vi "emi_Graph Background.vi"(0 "Graph Refnum":refnum<vi>, 1 "Width(Screen)":i32=-1, 2 "Height(Screen)":i32=-1, 3 "Dark(Black)":u32(colorbox), 4 "Light(White)":u32(colorbox)=16448250, 5 "error in":errorcluster, 6 "Graphic Type(FlatColor)":T1, 7 "Grid(Black)":u32(colorbox)) -> (14 "Graph Refnum Out":refnum<vi>, 19 "error out":errorcluster)   [LabVIEW 2011]
doc: "Set the background graphic for a graph. \nNote that With and height must be bigger then the largest size for the graph. If left blank, a background the size of the screen is generated.\nGrid is the color of the Major grid lines.\n\nSupported graphs:\nXYGraph\nDigitalGraph\nWaveform Graph\nMixedSignal Graph\n\nOn other graphs the background color will simply be set to the light color.\n\nOn error: No action performed"
uses:
  0 - General/Graphix/Private/emi_List Of Graphix.ctl
  <vilib>/picture/picture.llb/imagedata.ctl
  0 - General/Graphix/emi_BW 8Bit image to Linear DuoTone.vi
  0 - General/Graphix/emi_Tile Gradient Image.vi
  <vilib>/picture/picture.llb/Draw Flattened Pixmap.vi
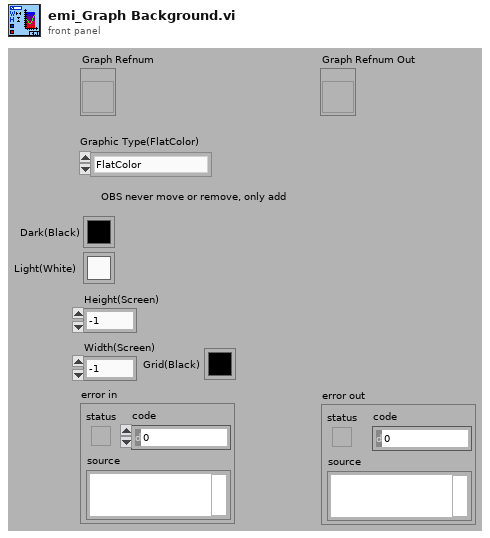
[diagram p1: front panel]
types:
  T1 = typedef "emi_List Of Graphix.ctl" = enum16{"FlatColor", "SharpGrad", "ShallowGrad", "GlasGradBord", "GlasGrad", "GlasGradBord 2"}
  T2 = typedef "imagedata.ctl" = cluster{"image type":i32, "image depth":i32, "image":u8[], "mask":u8[], "colors":u32[], "Rectangle":cluster{"left":i16, "top":i16, "right":i16, "bottom":i16}}
  T3 = typedef "LVRectTypeDef.ctl" = cluster{"left":i16, "top":i16, "right":i16, "bottom":i16}
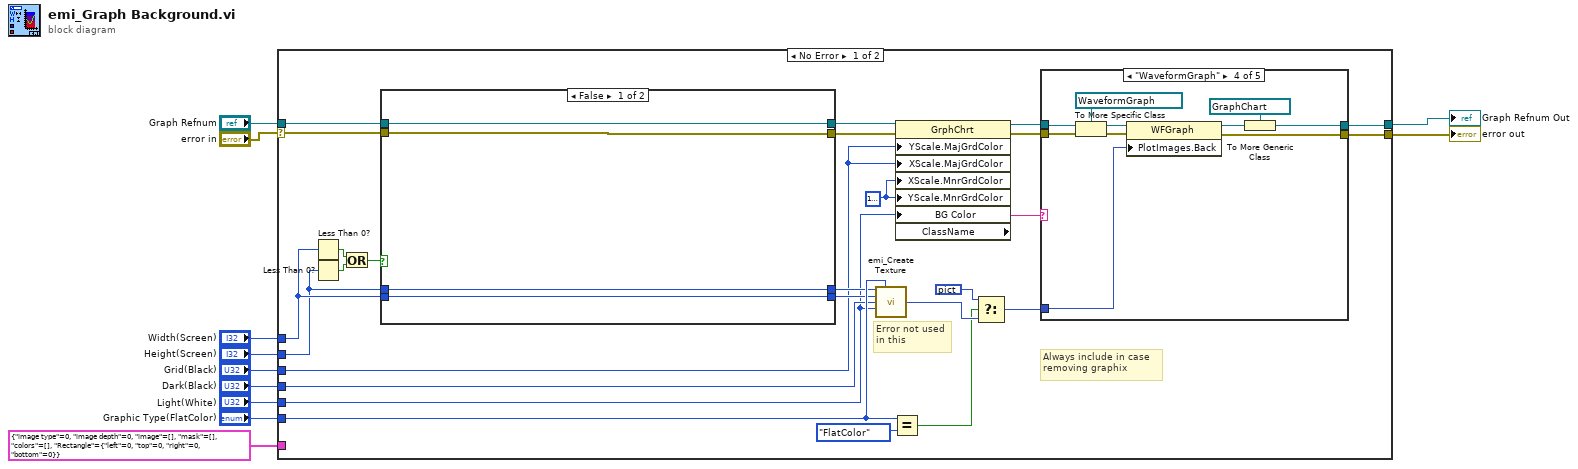
[diagram p0: block diagram]
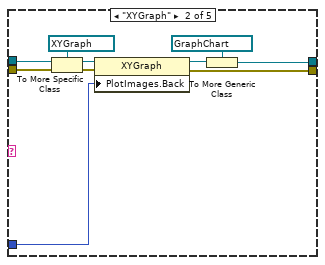
[diagram p3: hidden frame]
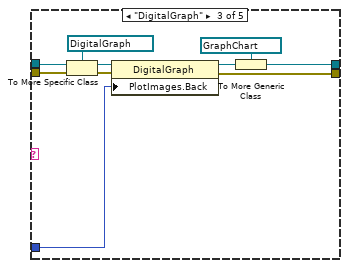
[diagram p4: hidden frame]
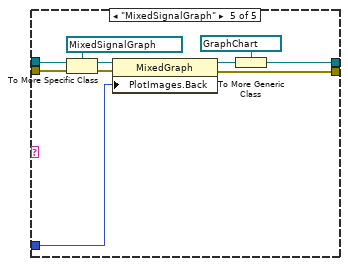
[diagram p5: hidden frame]
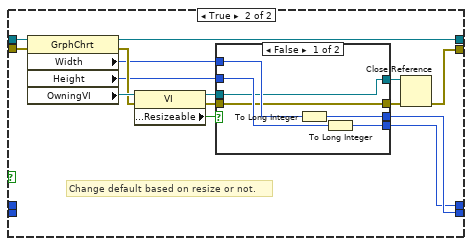
[diagram p6: hidden frame]
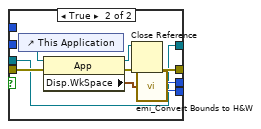
[diagram p7: hidden frame]
diagram:
  n1 = case shown="No Error" "error in" {
    selector: "error in" -> [w23 w115]
    tunnel: "Graphic Type(FlatColor)" -> [w36 _]
    tunnel: T2 {"image type"=0, "image depth"=0, "image"=[], "mask"=[], "colors"=[], "Rectangle"={"left"=0, "top"=0, "right"=0, "bottom"=0}} ("Image Data Out") -> [_ _]
    tunnel: "Graph Refnum" -> [w29 w114]
    tunnel: "Width(Screen)" -> [w26 _]
    tunnel: "Height(Screen)" -> [w25 _]
    tunnel: "Dark(Black)" -> [w20 _]
    tunnel: "Light(White)" -> [w13 _]
    tunnel: [w15 w115] -> w2
    tunnel: [w14 w114] -> w1
    tunnel: "Grid(Black)" -> [w12 _]
    frame No Error {
      w32 = u32 16777216 ("Light")
      # "Error not used\nin this"
      # "Always include in case\nremoving graphix"
      n2 = Less Than 0?(x=w26) -> (x < 0?=w30:bool)
      n3 = Less Than 0?(x=w25) -> (x < 0?=w31:bool)
      n4 = Or(x=w30, y=w31) -> (x .or. y?=w24:bool)
      n5 = case shown="False" w24 {
        tunnel: w29 -> [w83 w96]
        tunnel: [w83 w98] -> w28
        tunnel: w23 -> [w82 w97]
        tunnel: [w82 w86] -> w27
        tunnel: w26 -> [w80 _]
        tunnel: [w80 w89] -> w22
        tunnel: w25 -> [w81 _]
        tunnel: [w81 w88] -> w21
        frame False {
        }
        frame True {
          # "Change default based on resize or not."
          n6 = property class="GrphChrt"(reference=w96, error in=w97) -> (reference out=w98:refnum<vi>, error out=w94:errorcluster, "Width"=w91:u32, "Height"=w90:u32, "OwningVI"=w95:refnum<vi>)
          n7 = property class="VI"(reference=w95, error in=w94) -> (reference out=w85:refnum<vi>, error out=w93:errorcluster, "Front Panel.Resizeable"=w92:bool)
          n8 = case shown="False" w92 {
            tunnel: w93 -> [w102 w110]
            tunnel: [w102 w108] -> w87
            tunnel: w91 -> [w104 _]
            tunnel: w90 -> [w103 _]
            tunnel: [w100 w107] -> w89
            tunnel: [w99 w106] -> w88
            tunnel: w85 -> [w101 w105]
            tunnel: [w101 w105] -> w84
            frame False {
              n9 = To Long Integer(number=w104) -> (32bit integer=w100:i32)
              n10 = To Long Integer(number=w103) -> (32bit integer=w99:i32)
            }
            frame True {
              n11 = control-ref of="This Application"() -> (w109:refnum<vi>)
              n12 = property class="App"(reference=w109, error in=w110) -> (reference out=w112:refnum<vi>, error out=w113:errorcluster, "Disp.WkSpace"=w111:T3)
              n13 = Close Reference(reference=w112, error in (no error)=w113) -> (error out=w108:errorcluster)
              n14 = call "emi_Convert Bounds to H&W.vi"("Bounds"=w111) -> ("Width"=w107:i32, "Height"=w106:i32)  [unwired: 6 in]
            }
          }
          n15 = Close Reference(reference=w84, error in (no error)=w87) -> (error out=w86:errorcluster)
        }
      }
      n16 = call "emi_Create Texture.vi"("Height(600)"=w21, "Graphic Type(Flat Color)"=w36, "Width(400)"=w22, "Dark(Black)"=w20, "Light(White)"=w13) -> ("Picture Out"=w35:picture)  [unwired: 8 in, 2 out]
      n17 = Equal?(x=w36, y=emi_List_Of_Graphix."FlatColor" ("Graphic Type")) -> (x = y?=w33:bool)
      n18 = property class="GrphChrt"(reference=w28, error in=w27, "YScale.MajGrdColor"=w12, "XScale.MajGrdColor"=w12, "XScale.MnrGrdColor"=w32, "YScale.MnrGrdColor"=w32, "BG Color"=w13) -> (reference out=w19:refnum<vi>, error out=w16:errorcluster, "ClassName"=w17:string)
      n19 = Select(t=picture data[5B], s=w33, f=w35) -> (s? t:f=w18:picture)
      n20 = case shown="\"WaveformGraph\"" w17 {
        tunnel: w19 -> [w39 w48 w58 w68 w78]
        tunnel: w18 -> [_ w44 w54 w64 w74]
        tunnel: w16 -> [w38 w49 w59 w69 w79]
        tunnel: [w38 w40 w55 w65 w75] -> w15
        tunnel: [w39 w42 w50 w61 w71] -> w14
        frame "False", Default {
        }
        frame "XYGraph" {
          n21 = To More Specific Class(target class=refnum<vi> refnum ("XYGraph Refnum"), reference=w48, error in=w49) -> (specific class reference=w46:refnum<vi>, error out=w45:errorcluster)
          n22 = property class="XYGraph"(reference=w46, error in=w45, "PlotImages.Back"=w44) -> (reference out=w43:refnum<vi>, error out=w40:errorcluster)
          n23 = To More Generic Class(target class=refnum<vi> refnum ("GrphChrt Refnum"), reference=w43) -> (generic class reference=w42:refnum<vi>)
        }
        frame "DigitalGraph" {
          n24 = To More Specific Class(target class=refnum<vi> refnum ("DigitalGraph Refnum"), reference=w58, error in=w59) -> (specific class reference=w57:refnum<vi>, error out=w56:errorcluster)
          n25 = property class="DigitalGraph"(reference=w57, error in=w56, "PlotImages.Back"=w54) -> (reference out=w51:refnum<vi>, error out=w55:errorcluster)
          n26 = To More Generic Class(target class=refnum<vi> refnum ("GrphChrt Refnum"), reference=w51) -> (generic class reference=w50:refnum<vi>)
        }
        frame "WaveformGraph" {
          n27 = To More Specific Class(target class=refnum<vi> refnum ("WFGraph Refnum"), reference=w68, error in=w69) -> (specific class reference=w67:refnum<vi>, error out=w66:errorcluster)
          n28 = property class="WFGraph"(reference=w67, error in=w66, "PlotImages.Back"=w64) -> (reference out=w62:refnum<vi>, error out=w65:errorcluster)
          n29 = To More Generic Class(target class=refnum<vi> refnum ("GrphChrt Refnum"), reference=w62) -> (generic class reference=w61:refnum<vi>)
        }
        frame "MixedSignalGraph" {
          n30 = To More Specific Class(target class=refnum<vi> refnum ("MixedGraph Refnum"), reference=w78, error in=w79) -> (specific class reference=w77:refnum<vi>, error out=w76:errorcluster)
          n31 = property class="MixedGraph"(reference=w77, error in=w76, "PlotImages.Back"=w74) -> (reference out=w72:refnum<vi>, error out=w75:errorcluster)
          n32 = To More Generic Class(target class=refnum<vi> refnum ("GrphChrt Refnum"), reference=w72) -> (generic class reference=w71:refnum<vi>)
        }
      }
    }
    frame Error {
    }
  }
  "error out" <- w2
  "Graph Refnum Out" <- w1
